vi "VEHICLE.vi"() -> ()   [LabVIEW 2020]
uses:
  <vilib>/Utility/file.llb/Write Delimited Spreadsheet (string).vi
panel:
  in  "?":bool
  in  "BOOTH NO":string(combo)
  out "PAYMENT PROCESS":bool
  in  "?":bool
  in  "PASSWORD":string
  in  "CASH PAYMENT":string(combo)
  out "TWO WAY":bool
  out "ONE WAY":bool
  in  "WAY":bool
  in  "OPERATOR NAME":string
  out "DISPLAY":string
  in  "VEHICLE TYPE":string(combo)
  in  "VEHICLE NO":string
  out "GATE STATUS":bool
  in  "?":bool
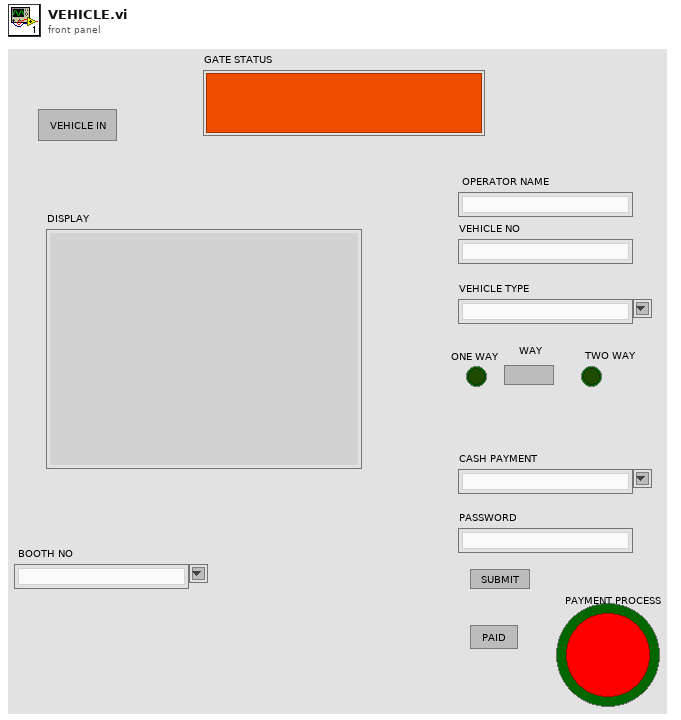
[diagram p1: front panel]
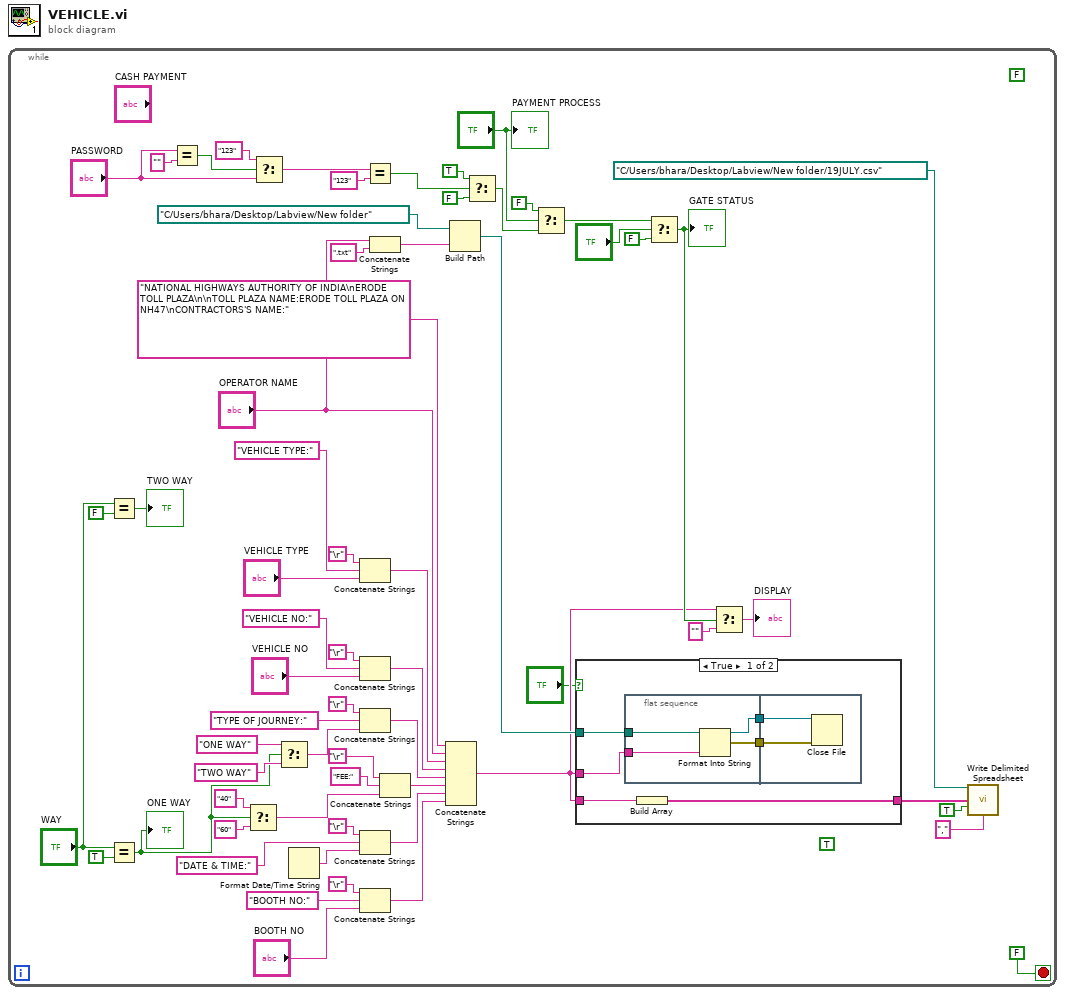
[diagram p0: block diagram]
diagram:
  n1 = while {
    stop <- FALSE stop-if-true
    (unwired) TRUE ("y")
    (unwired) FALSE ("y")
    n2 = Equal?(x="WAY", y=FALSE) -> (x = y?=→"TWO WAY":bool)
    n3 = Equal?(x="WAY", y=TRUE) -> (x = y?=w37:bool)
    "ONE WAY" <- w37
    n4 = Equal?(x="PASSWORD", y="") -> (x = y?=w29:bool)
    n5 = Select(t="40", s=w37, f="60") -> (s? t:f=w59:string)
    n6 = Select(t="123", s=w29, f="PASSWORD") -> (s? t:f=w26:string)
    n7 = Select(t="ONE WAY", s=w37, f="TWO WAY") -> (s? t:f=w55:string)
    n8 = Format Date/Time String() -> (date/time string=w6:string)  [unwired: 3 in]
    n9 = Concatenate Strings("\r" ("string"), "VEHICLE TYPE:" ("string"), "VEHICLE TYPE") -> (w42:string)
    n10 = Concatenate Strings("\r" ("string"), "VEHICLE NO:" ("string"), "VEHICLE NO") -> (w46:string)
    n11 = Concatenate Strings("\r" ("string"), "TYPE OF JOURNEY:" ("string"), w55) -> (w41:string)
    n12 = Concatenate Strings("\r" ("string"), "DATE & TIME:" ("string"), w6) -> (w39:string)
    n13 = Concatenate Strings("\r" ("string"), "BOOTH NO:" ("string"), "BOOTH NO") -> (w10:string)
    n14 = Equal?(x=w26, y="123") -> (x = y?=w31:bool)
    n15 = Concatenate Strings("OPERATOR NAME", ".txt" ("string")) -> (w18:string)
    n16 = Concatenate Strings("\r" ("string"), "FEE:" ("string"), w59) -> (w40:string)
    n17 = Concatenate Strings("NATIONAL HIGHWAYS AUTHORITY OF INDIA\nERODE TOLL PLAZA\n\nTOLL PLAZA NAME:ERODE TOLL PLAZA ON NH47\nCONTRACTORS'S NAME:" ("string"), "OPERATOR NAME", w42, w46, w41, w40, w39, w10) -> (w8:string)
    n18 = Build Path(base path=path "C:/Users/bhara/Desktop/Labview/New folder", name or relative path=w18) -> (appended path=w16:path)
    n19 = Select(t=TRUE, s=w31, f=FALSE) -> (s? t:f=w14:bool)
    n20 = Select(t=FALSE, s="?", f=w14) -> (s? t:f=w12:bool)
    n21 = case shown="True" "?" {
      tunnel: w8 -> [w67 _]
      tunnel: w16 -> [w70 _]
      tunnel: w8 -> [w66 _]
      tunnel: [w65 _] -> w3
      frame True {
        n22 = flat-sequence {
          tunnel: w67 -> [w74]
          tunnel: w70 -> [w73]
          tunnel: [w72] -> w69
          tunnel: [w71] -> w68
          tunnel: w69 -> [w76]
          tunnel: w68 -> [w75]
          frame #0 {
            n23 = Format Into String(initial string=w73, w74) -> (resulting string=w72:refnum<file>, error out=w71:errorcluster)  [unwired: 2 in]
          }
          frame #1 {
            n24 = Close File(refnum=w76, error in=w75) -> ()  [unwired: 2 out]
          }
        }
        n25 = Build Array(w66) -> (w65:string[])
      }
      frame False {
      }
    }
    n26 = Select(t=w12, s="?", f=FALSE) -> (s? t:f=w21:bool)
    "GATE STATUS" <- w21
    n27 = Select(t=w8, s=w21, f="") -> (s? t:f=→"DISPLAY":string)
    n28 = call-poly <vilib>:"Write Delimited Spreadsheet.vi"("file path (dialog if empty)"=path "C:/Users/bhara/Desktop/Labview/New folder/19JULY.csv" ("base path"), "1D data"=w3, "append to file? (new file:F)"=TRUE, "delimiter (\\t)"="," ("delimiter (\\t)")) -> ()  [unwired: 10 in, 2 out]
    "PAYMENT PROCESS" <- "?"
  }
